vi "read_data_linear_z_mt_connect (SubVI).vi"(8 "error in (no error)":errorcluster, 11 "URL":string="http://amrcadp:5000/current?&path=//") -> (0 "error out":errorcluster, 3 "number":dbl[](array[numeric]))   [LabVIEW 2017]
uses:
  <vilib>/xml/Load XML String.vi
  <vilib>/xml/Close Reference(Node).vi
  <vilib>/addons/internet/NI_InternetTK_Core_VIs.lvlib
  <vilib>/xml/NI_XML.lvlib
  <resource>/objmgr/DOMUserDefRef.rc
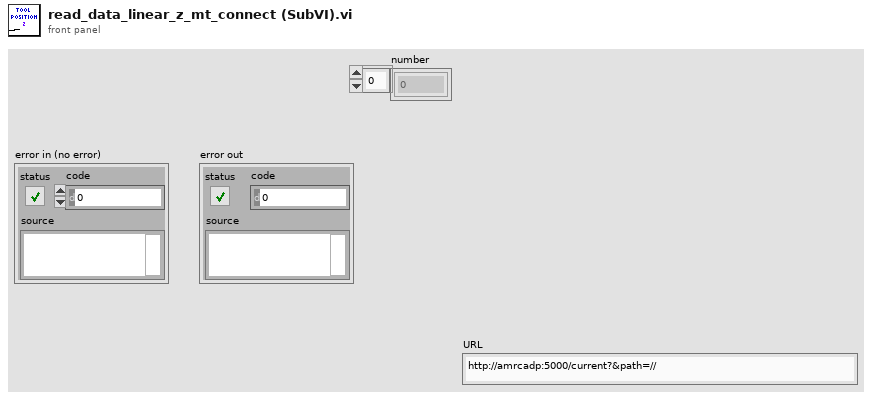
[diagram p1: front panel]
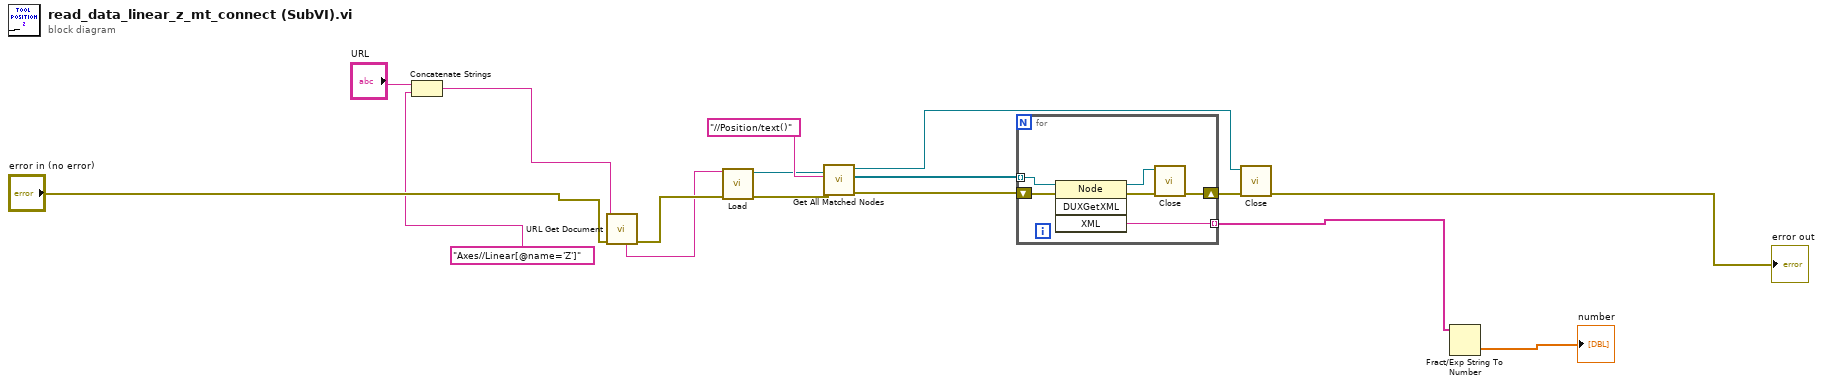
[diagram p0: block diagram]
diagram:
  n1 = Concatenate Strings("URL", "Axes//Linear[@name='Z']" ("URL")) -> (w1:string)
  n2 = call <vilib>:"URL Get Document.vi"("error in (no error)"="error in (no error)", "URL"=w1) -> ("error out"=w14:errorcluster, "content"=w12:string)  [unwired: 5 in, 3 out]
  n3 = call-poly <vilib>:"Load.vi"("XML string"=w12, "error in (no error)"=w14) -> ("DOM document out"=w9:refnum<k20>, "error out"=w10:errorcluster)  [unwired: 11 in, 1 out]
  n4 = call <vilib>:"Get All Matched Nodes.vi"("error in (no error)"=w10, "XPath expression"="//Position/text()", "node in"=w9) -> ("error out"=w7:errorcluster, "node result array"=w6:refnum<k20>[], "node out"=w11:refnum<k20>)  [unwired: 6 out]
  n5 = for {
    tunnel: w6 -> [w18] mode=indexing
    shift-right: [w20] -> w8
    shift-left: w7 -> [w19]
    tunnel: [w17] -> w5 mode=indexing
    n6 = invoke on="Invoke Node" class="Node" method="DUXGetXML"(reference=w18, error in=w19) -> (reference out=w21:refnum<k20>, error out=w22:errorcluster, "XML"=w17:string)  [unwired: 2 in, 1 out]
    n7 = call-poly <vilib>:"Close.vi"("error in (no error)"=w22, "node"=w21) -> ("error out"=w20:errorcluster)  [unwired: 7 out]
  }
  n8 = call-poly <vilib>:"Close.vi"("error in (no error)"=w8, "node"=w11) -> ("error out"=→"error out":errorcluster)  [unwired: 7 out]
  n9 = Fract/Exp String To Number(string=w5) -> (number=→"number":dbl[])  [unwired: 3 in, 1 out]
